vi "Get Rectangle Corners.vi"(0 "Rect Data":T2) -> (1 "Top Left":cluster{"X":dbl, "Y":dbl}, 2 "Top Right":cluster{"X":dbl, "Y":dbl}, 3 "Bottom Right":cluster{"X":dbl, "Y":dbl}, 4 "Bottom Left":cluster{"X":dbl, "Y":dbl})   [LabVIEW 2019]
doc: "This VI retrieves the corners of a rectangle from the Inkscape data."
uses:
  <vilib>/Analysis/Matrix/Datatypes/RealMatrix.ctl
  <vilib>/Analysis/Matrix/NI_Matrix.lvlib
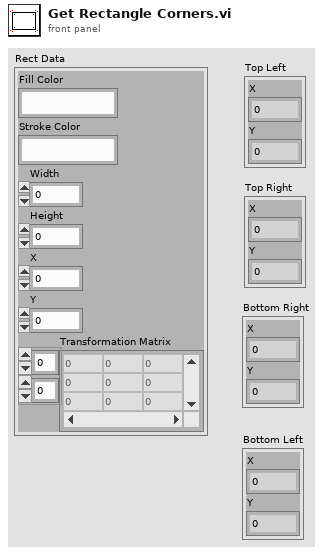
[diagram p1: front panel]
types:
  T1 = typedef "NI_Matrix.lvlib/RealMatrix.ctl" = dbl[][]
  T2 = cluster{"Fill Color":string, "Stroke Color":string, "Width":dbl, "Height":dbl, "X":dbl, "Y":dbl, "Transformation Matrix":T1}
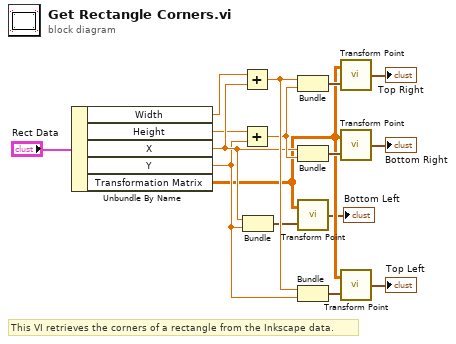
[diagram p0: block diagram]
diagram:
  # "This VI retrieves the corners of a rectangle from the Inkscape data."
  n1 = Unbundle By Name("Rect Data") -> ("Width"=w14:dbl, "Height"=w11:dbl, "X"=w13:dbl, "Y"=w12:dbl, "Transformation Matrix"=w2:T1)
  n2 = Add(x=w14, y=w13) -> (x+y=w16:dbl)
  n3 = Add(x=w11, y=w12) -> (x+y=w15:dbl)
  n4 = Bundle("X"=w13, "Y"=w12) -> (w3:cluster{"X":dbl, "Y":dbl})  [unwired: 1 in]
  n5 = Bundle(w16, w15) -> (w7:cluster{dbl, dbl})  [unwired: 1 in]
  n6 = Bundle("X"=w13, w15) -> (w5:cluster{"X":dbl, dbl})  [unwired: 1 in]
  n7 = call "Transform Point.vi"("Point to Transform"=w3, "Transformation Matrix"=w2) -> ("Transformed Point"=→"Bottom Left":cluster{"X":dbl, "Y":dbl})
  n8 = Bundle(w16, "Y"=w12) -> (w9:cluster{dbl, "Y":dbl})  [unwired: 1 in]
  n9 = call "Transform Point.vi"("Point to Transform"=w7, "Transformation Matrix"=w2) -> ("Transformed Point"=→"Top Right":cluster{"X":dbl, "Y":dbl})
  n10 = call "Transform Point.vi"("Point to Transform"=w5, "Transformation Matrix"=w2) -> ("Transformed Point"=→"Bottom Right":cluster{"X":dbl, "Y":dbl})
  n11 = call "Transform Point.vi"("Point to Transform"=w9, "Transformation Matrix"=w2) -> ("Transformed Point"=→"Top Left":cluster{"X":dbl, "Y":dbl})
